vi "BRig_dataExp_I_Cue2.vi"() -> (2 "output_I_Cue2":i32)   [LabVIEW 2014]
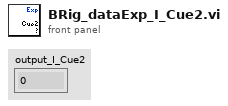
[diagram p1: front panel]
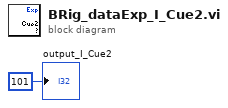
[diagram p0: block diagram]
diagram:
  "output_I_Cue2" <- 101 ("output_iBlock")
